vi "Lab 1 Part b.vi"() -> ()   [LabVIEW 2024]
panel:
  in  "stop":bool
  out "X * X":dbl
  in  "X":dbl
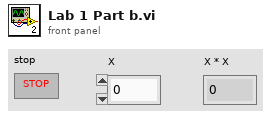
[diagram p1: front panel]
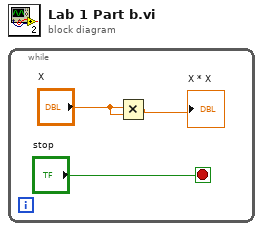
[diagram p0: block diagram]
diagram:
  n1 = while {
    stop <- "stop" stop-if-true
    n2 = Multiply(x="X", y="X") -> (x*y=→"X * X":dbl)
  }
